vi "Find Lines.vi"(11 "Filtered Targets":T4[](array[typedef])) -> (2 "Diamond Targets":T1[](array[typedef]), 3 "Lines":T5[][](array[typedef]))   [LabVIEW 2011]
uses:
  Line.ctl
  Direction.ctl
  Line Confidence.ctl
  Target.ctl
  Diamond Target Output.ctl
  Rectangle Position.ctl
  Target Confidence.ctl
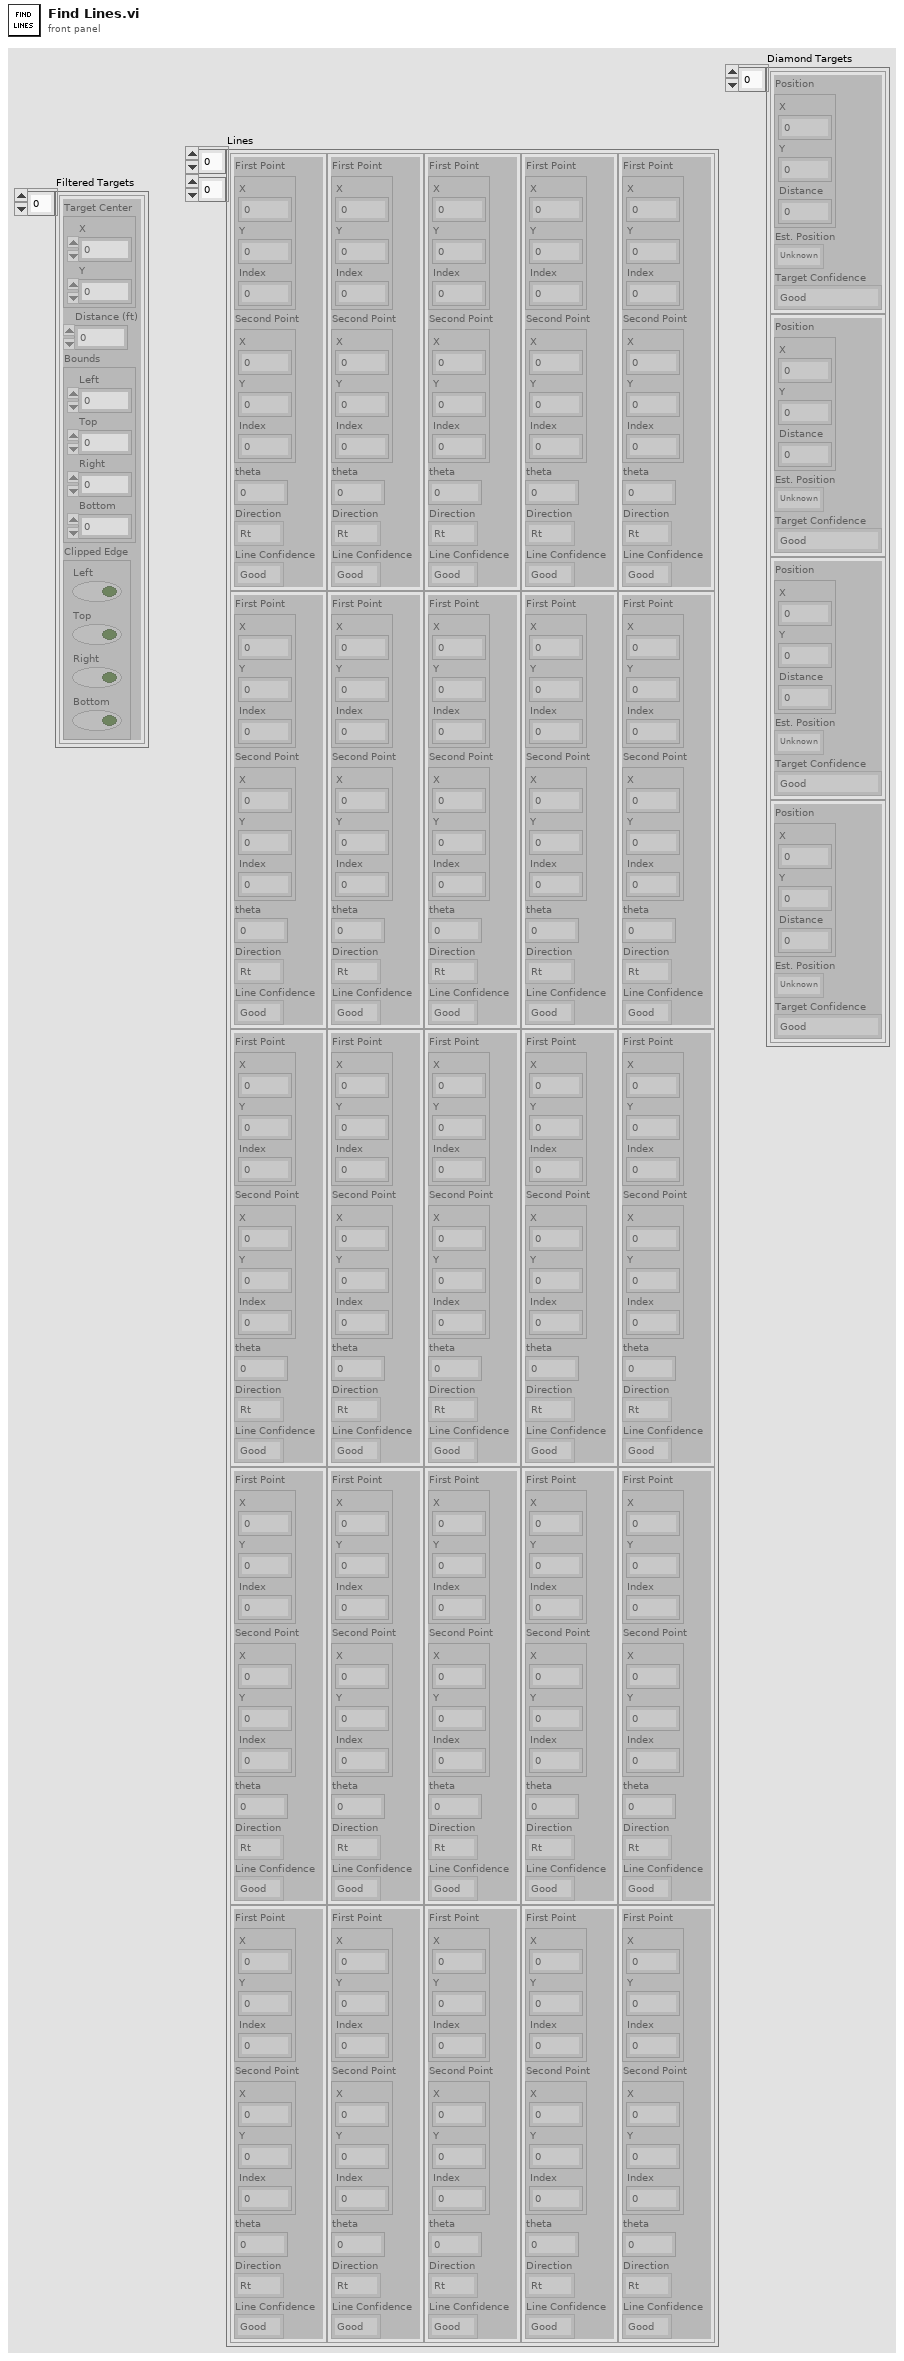
[diagram p1: front panel]
types:
  T1 = typedef "Diamond Target Output.ctl" = cluster{"Position":cluster{"X":dbl, "Y":dbl, "Distance":dbl}, "Est. Position":T2, "Target Confidence":T3}
  T2 = typedef "Rectangle Position.ctl" = enum16{"Unknown", "Top", "Right", "Left", "Bottom"}
  T3 = typedef "Target Confidence.ctl" = enum16{"Good", "Good-Clipped Y", "Marginal-Clipped X"}
  T4 = typedef "Target.ctl" = cluster{"Target Center":cluster{"X":dbl, "Y":dbl}, "Distance (ft)":dbl, "Bounds":cluster{"Left":dbl, "Top":dbl, "Right":dbl, "Bottom":dbl}, "Clipped Edge":cluster{"Left":bool, "Top":bool, "Right":bool, "Bottom":bool}}
  T5 = typedef "Line.ctl" = cluster{"First Point":cluster{"X":dbl, "Y":dbl, "Index":dbl}, "Second Point":cluster{"X":dbl, "Y":dbl, "Index":dbl}, "theta":dbl, "Direction":T6, "Line Confidence":T7}
  T6 = typedef "Direction.ctl" = enum16{"Rt", "Rt-Up", "Up", "Lt-Up", "Lt", "Lt-Dn", "Dn", "Rt-Dn", "Unknown"}
  T7 = typedef "Line Confidence.ctl" = enum16{"Good", "Bad"}
  T8 = cluster{"Left":bool, "Top":bool, "Right":bool, "Bottom":bool}
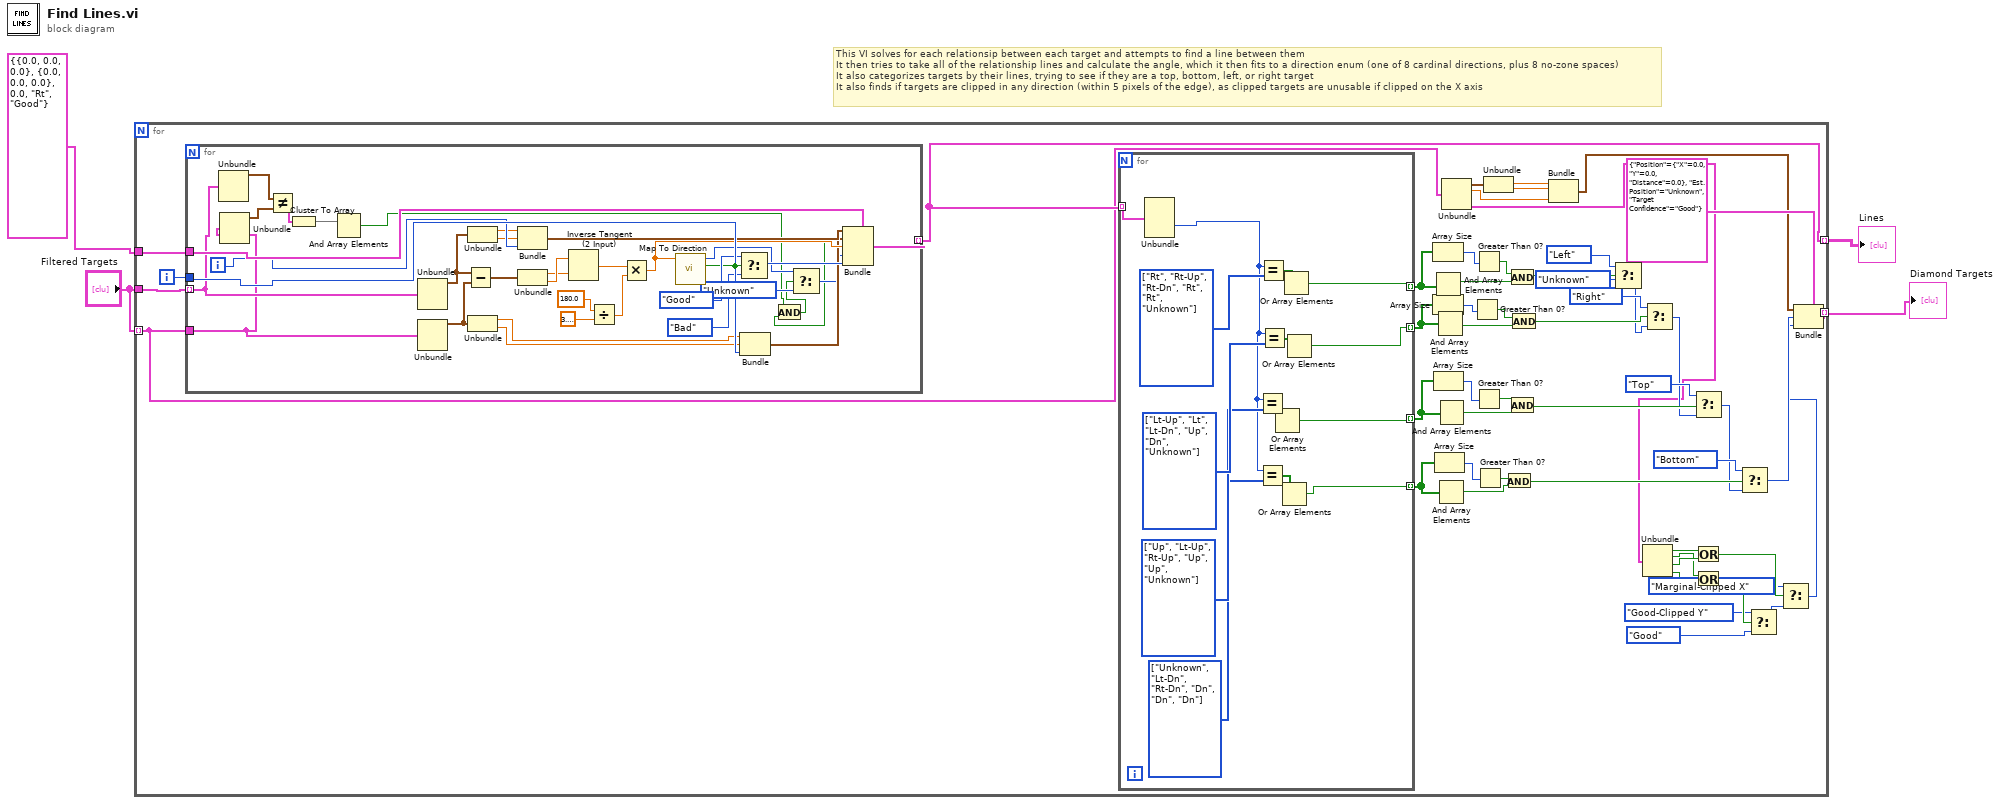
[diagram p0: block diagram]
diagram:
  # "This VI solves for each relationsip between each target and attempts to find a line between them\nIt then tries to take all of the relationship lines and calculate the angle, which it then fits to a direction enum (one of 8 cardinal directions, plus 8 no-zone spaces)\nIt also categorizes targets by their lines, trying to see if they are a top, bottom, left, or right target\nIt also finds if targets are clipped in any direction (within 5 pixels of the edge), as clipped targets are unusable if clipped on the X axis"
  n1 = for {
    tunnel: "Filtered Targets" -> [w23] mode=indexing
    tunnel: "Filtered Targets" -> [w24]
    tunnel: T5 {"First Point"={"X"=0.0, "Y"=0.0, "Index"=0.0}, "Second Point"={"X"=0.0, "Y"=0.0, "Index"=0.0}, "theta"=0.0, "Direction"=enum."Rt", "Line Confidence"=enum."Good"} ("Line") -> [w56]
    tunnel: [w25] -> w4 mode=indexing
    tunnel: [w22] -> w1 mode=indexing
    i -> [w57]
    n2 = for {
      tunnel: w23 -> [w102]
      tunnel: w24 -> [w103] mode=indexing
      tunnel: w57 -> [w105]
      tunnel: w56 -> [w106]
      tunnel: [w78] -> w25 mode=indexing
      i -> [w104]
      n3 = Unbundle(w103) -> ("Target Center"=w101:cluster{"X":dbl, "Y":dbl})  [unwired: 3 out]
      n4 = Unbundle(w102) -> ("Target Center"=w100:cluster{"X":dbl, "Y":dbl})  [unwired: 3 out]
      n5 = Not Equal?(x=w101, y=w100) -> (x != y?=w99:cluster{"X":bool, "Y":bool})
      n6 = Cluster To Array(cluster=w99) -> (array=w98:bool[])
      n7 = And Array Elements(Boolean array=w98) -> (logical AND=w73:bool)
      n8 = Unbundle(w103) -> ("Target Center"=w79:cluster{"X":dbl, "Y":dbl})  [unwired: 3 out]
      n9 = Unbundle(w102) -> ("Target Center"=w80:cluster{"X":dbl, "Y":dbl})  [unwired: 3 out]
      n10 = Subtract(x=w79, y=w80) -> (x-y=w97:cluster{"X":dbl, "Y":dbl})
      n11 = Unbundle(w79) -> ("X"=w84:dbl, "Y"=w83:dbl)
      n12 = Unbundle(w80) -> ("X"=w86:dbl, "Y"=w85:dbl)
      n13 = Bundle("X"=w84, "Y"=w83, w104) -> (w82:cluster{"X":dbl, "Y":dbl, i32})  [unwired: 1 in]
      n14 = Unbundle(w97) -> ("X"=w95:dbl, "Y"=w96:dbl)
      n15 = Inverse Tangent (2 Input)(1:w95, 2:w96) -> (0:w94:dbl)
      n16 = Divide(x=180.0, y=3.141592653589793) -> (x/y=w93:dbl)
      n17 = Multiply(x=w94, y=w93) -> (x*y=w90:dbl)
      n18 = call "Map To Direction.vi"("Theta"=w90) -> ("In Range?"=w72:bool, "Direction"=w76:T6)  [unwired: 9 in]
      n19 = Select(t=Line_Confidence."Good" ("Line Confidence"), s=w72, f=Line_Confidence."Bad") -> (s? t:f=w88:T7)
      n20 = Bundle("X"=w86, "Y"=w85, w105) -> (w81:cluster{"X":dbl, "Y":dbl, i32})  [unwired: 1 in]
      n21 = And(x=w73, y=w72) -> (x .and. y?=w74:bool)
      n22 = Select(t=w76, s=w74, f=Direction."Unknown") -> (s? t:f=w77:T6)
      n23 = Bundle(cluster=w106, "First Point"=w82, "Second Point"=w81, "theta"=w90, "Direction"=w77, "Line Confidence"=w88) -> (w78:T5)
    }
    n24 = for {
      tunnel: w25 -> [w71] mode=indexing
      tunnel: [w58] -> w51 mode=indexing
      tunnel: [w59] -> w50 mode=indexing
      tunnel: [w60] -> w49 mode=indexing
      tunnel: [w61] -> w48 mode=indexing
      w67 = T6[] [enum."Unknown", enum."Lt-Dn", enum."Rt-Dn", enum."Dn", enum."Dn", enum."Dn"] items=["Rt", "Rt-Up", "Up", "Lt-Up", "Lt", "Lt-Dn", "Dn", "Rt-Dn", "Unknown"]
      w68 = T6[] [enum."Up", enum."Lt-Up", enum."Rt-Up", enum."Up", enum."Up", enum."Unknown"] items=["Rt", "Rt-Up", "Up", "Lt-Up", "Lt", "Lt-Dn", "Dn", "Rt-Dn", "Unknown"]
      w69 = T6[] [enum."Lt-Up", enum."Lt", enum."Lt-Dn", enum."Up", enum."Dn", enum."Unknown"] items=["Rt", "Rt-Up", "Up", "Lt-Up", "Lt", "Lt-Dn", "Dn", "Rt-Dn", "Unknown"]
      w70 = T6[] [enum."Rt", enum."Rt-Up", enum."Rt-Dn", enum."Rt", enum."Rt", enum."Unknown"] items=["Rt", "Rt-Up", "Up", "Lt-Up", "Lt", "Lt-Dn", "Dn", "Rt-Dn", "Unknown"]
      n25 = Unbundle(w71) -> ("Direction"=w66:T6)  [unwired: 4 out]
      n26 = Equal?(x=w66, y=w68) -> (x = y?=w63:bool[])
      n27 = Equal?(x=w66, y=w67) -> (x = y?=w62:bool[])
      n28 = Equal?(x=w66, y=w70) -> (x = y?=w65:bool[])
      n29 = Equal?(x=w66, y=w69) -> (x = y?=w64:bool[])
      n30 = Or Array Elements(Boolean array=w63) -> (logical OR=w60:bool)
      n31 = Or Array Elements(Boolean array=w62) -> (logical OR=w61:bool)
      n32 = Or Array Elements(Boolean array=w65) -> (logical OR=w58:bool)
      n33 = Or Array Elements(Boolean array=w64) -> (logical OR=w59:bool)
    }
    n34 = Array Size(array=w51) -> (size(s)=w46:i32)
    n35 = And Array Elements(Boolean array=w51) -> (logical AND=w55:bool)
    n36 = Array Size(array=w50) -> (size(s)=w44:i32)
    n37 = Array Size(array=w49) -> (size(s)=w42:i32)
    n38 = And Array Elements(Boolean array=w50) -> (logical AND=w54:bool)
    n39 = Array Size(array=w48) -> (size(s)=w41:i32)
    n40 = And Array Elements(Boolean array=w48) -> (logical AND=w52:bool)
    n41 = And Array Elements(Boolean array=w49) -> (logical AND=w53:bool)
    n42 = Unbundle(w23) -> ("Target Center"=w9:cluster{"X":dbl, "Y":dbl}, "Distance (ft)"=w5:dbl, "Clipped Edge"=w21:T8)  [unwired: 1 out]
    n43 = Greater Than 0?(x=w44) -> (x > 0?=w45:bool)
    n44 = Greater Than 0?(x=w46) -> (x > 0?=w47:bool)
    n45 = Greater Than 0?(x=w42) -> (x > 0?=w43:bool)
    n46 = Greater Than 0?(x=w41) -> (x > 0?=w40:bool)
    n47 = Unbundle(w9) -> ("X"=w7:dbl, "Y"=w6:dbl)
    n48 = And(x=w40, y=w52) -> (x .and. y?=w33:bool)
    n49 = And(x=w47, y=w55) -> (x .and. y?=w39:bool)
    n50 = And(x=w43, y=w53) -> (x .and. y?=w35:bool)
    n51 = And(x=w45, y=w54) -> (x .and. y?=w37:bool)
    n52 = Bundle("X"=w7, "Y"=w6, "Distance (ft)"=w5) -> (w8:cluster{"X":dbl, "Y":dbl, "Distance (ft)":dbl})  [unwired: 1 in]
    n53 = Select(t=Rectangle_Position."Left" ("Rectangle Position"), s=w39, f=Rectangle_Position."Unknown") -> (s? t:f=w30:T2)
    n54 = Unbundle(w21) -> ("Left"=w20:bool, "Top"=w18:bool, "Right"=w19:bool, "Bottom"=w17:bool)
    n55 = Select(t=Rectangle_Position."Right" ("Rectangle Position"), s=w37, f=w30) -> (s? t:f=w31:T2)
    n56 = Select(t=Rectangle_Position."Top" ("Rectangle Position"), s=w35, f=w31) -> (s? t:f=w32:T2)
    n57 = Or(x=w20, y=w19) -> (x .or. y?=w12:bool)
    n58 = Or(x=w18, y=w17) -> (x .or. y?=w15:bool)
    n59 = Select(t=Rectangle_Position."Bottom" ("Rectangle Position"), s=w33, f=w32) -> (s? t:f=w26:T2)
    n60 = Select(t=Target_Confidence."Good-Clipped Y", s=w15, f=Target_Confidence."Good" ("Target Confidence")) -> (s? t:f=w13:T3)
    n61 = Select(t=Target_Confidence."Marginal-Clipped X", s=w12, f=w13) -> (s? t:f=w10:T3)
    n62 = Bundle(cluster=T1 {"Position"={"X"=0.0, "Y"=0.0, "Distance"=0.0}, "Est. Position"=enum."Unknown", "Target Confidence"=enum."Good"} ("Diamond Target Type"), "Position"=w8, "Est. Position"=w26, "Target Confidence"=w10) -> (w22:T1)
  }
  "Lines" <- w4
  "Diamond Targets" <- w1
